vi "shag_start — 4.vi"() -> ()   [LabVIEW 2016]
uses:
  <vilib>/Instr/_visa.llb/VISA Configure Serial Port (Instr).vi
panel:
  out "положение в мин 1":i32
  in  "stop":bool
  in  "all":T1(tab)
  out "положение шд":i32(knob) scale=-10.0..190.0
  out "текущее положение":string
  out "положение в минутах 1":string
  in  "Минуты":i32 min=-600 max=11400
  in  "Stop двигатель":bool
  in  "Вращение по градусам +":bool
  in  "Вращение по градусам -":bool
  in  "Вернуться в нулевое положение":bool
  in  "Задать текущее положение нулевым":bool
  in  "Установка минут":bool
  in  "Блокировать зеркало №1":bool
  in  "Выберете COM порт":refnum<visa-resource-name>="COM1"
  in  "Скорость обмена данными":u32(ring)=19200 items=["9600"=9600, "19200"=19200, "38400"=38400, "57600"=57600]
  in  "Число бит на символ":u16=8 min=5 max=8 step=1
  in  "Контроль чётности":enum16{"None", "Odd", "Even", "Mark", "Space"}(ring)
  in  "Стоповый бит":u16(ring)=10 items=["1.0"=10, "1.5"=15, "2.0"=20]
  in  "Контроль переполнения":u16(ring) items=["None"=0, "XON/XOFF"=1, "RTS/CTS"=2, "DTR/DSR"=4]
  # "1 - адресс 1 двигателя\n2 - адресс 2 двигателя\n$0MV\\01+   - запуск всех двигателей в положительном направлении \n$0MS\\00   - остановка всех двигателей\n$0MJ\\04+\\00\\00\\01   - 1 шаг всех двигателей\n$0SS\\01\\10   - скорость 10 для всех двигателей"
  # "Зеркало №1:"
  # "Положение:"
  # "Ренгеновская трубка №2:"
  # "Положение ренгеновской трубк:"
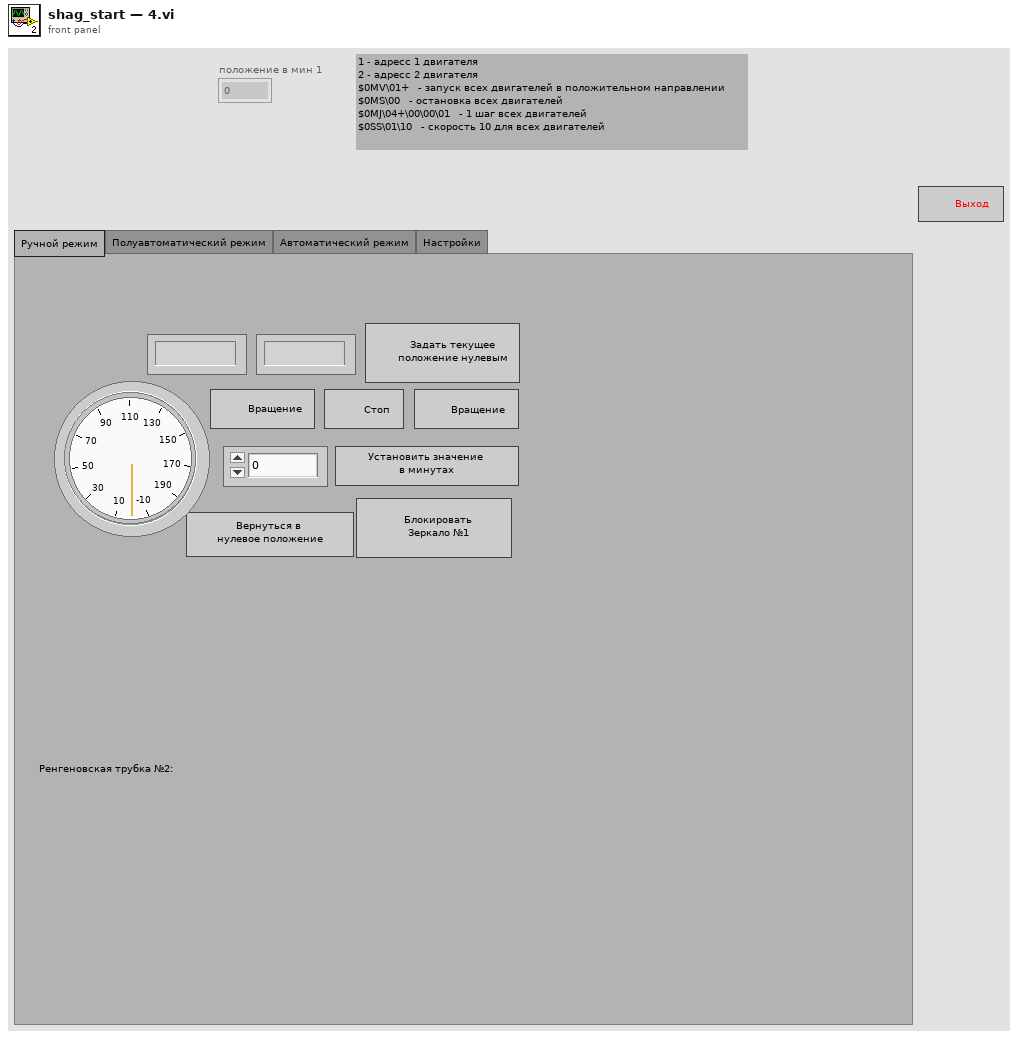
[diagram p1: front panel]
types:
  T1 = enum32{"Ручной режим", "Полуавтоматический режим", "Автоматический режим", "Настройки"}
  T2 = enum8{"Enabled", "Disabled", "Disabled and Grayed Out"}
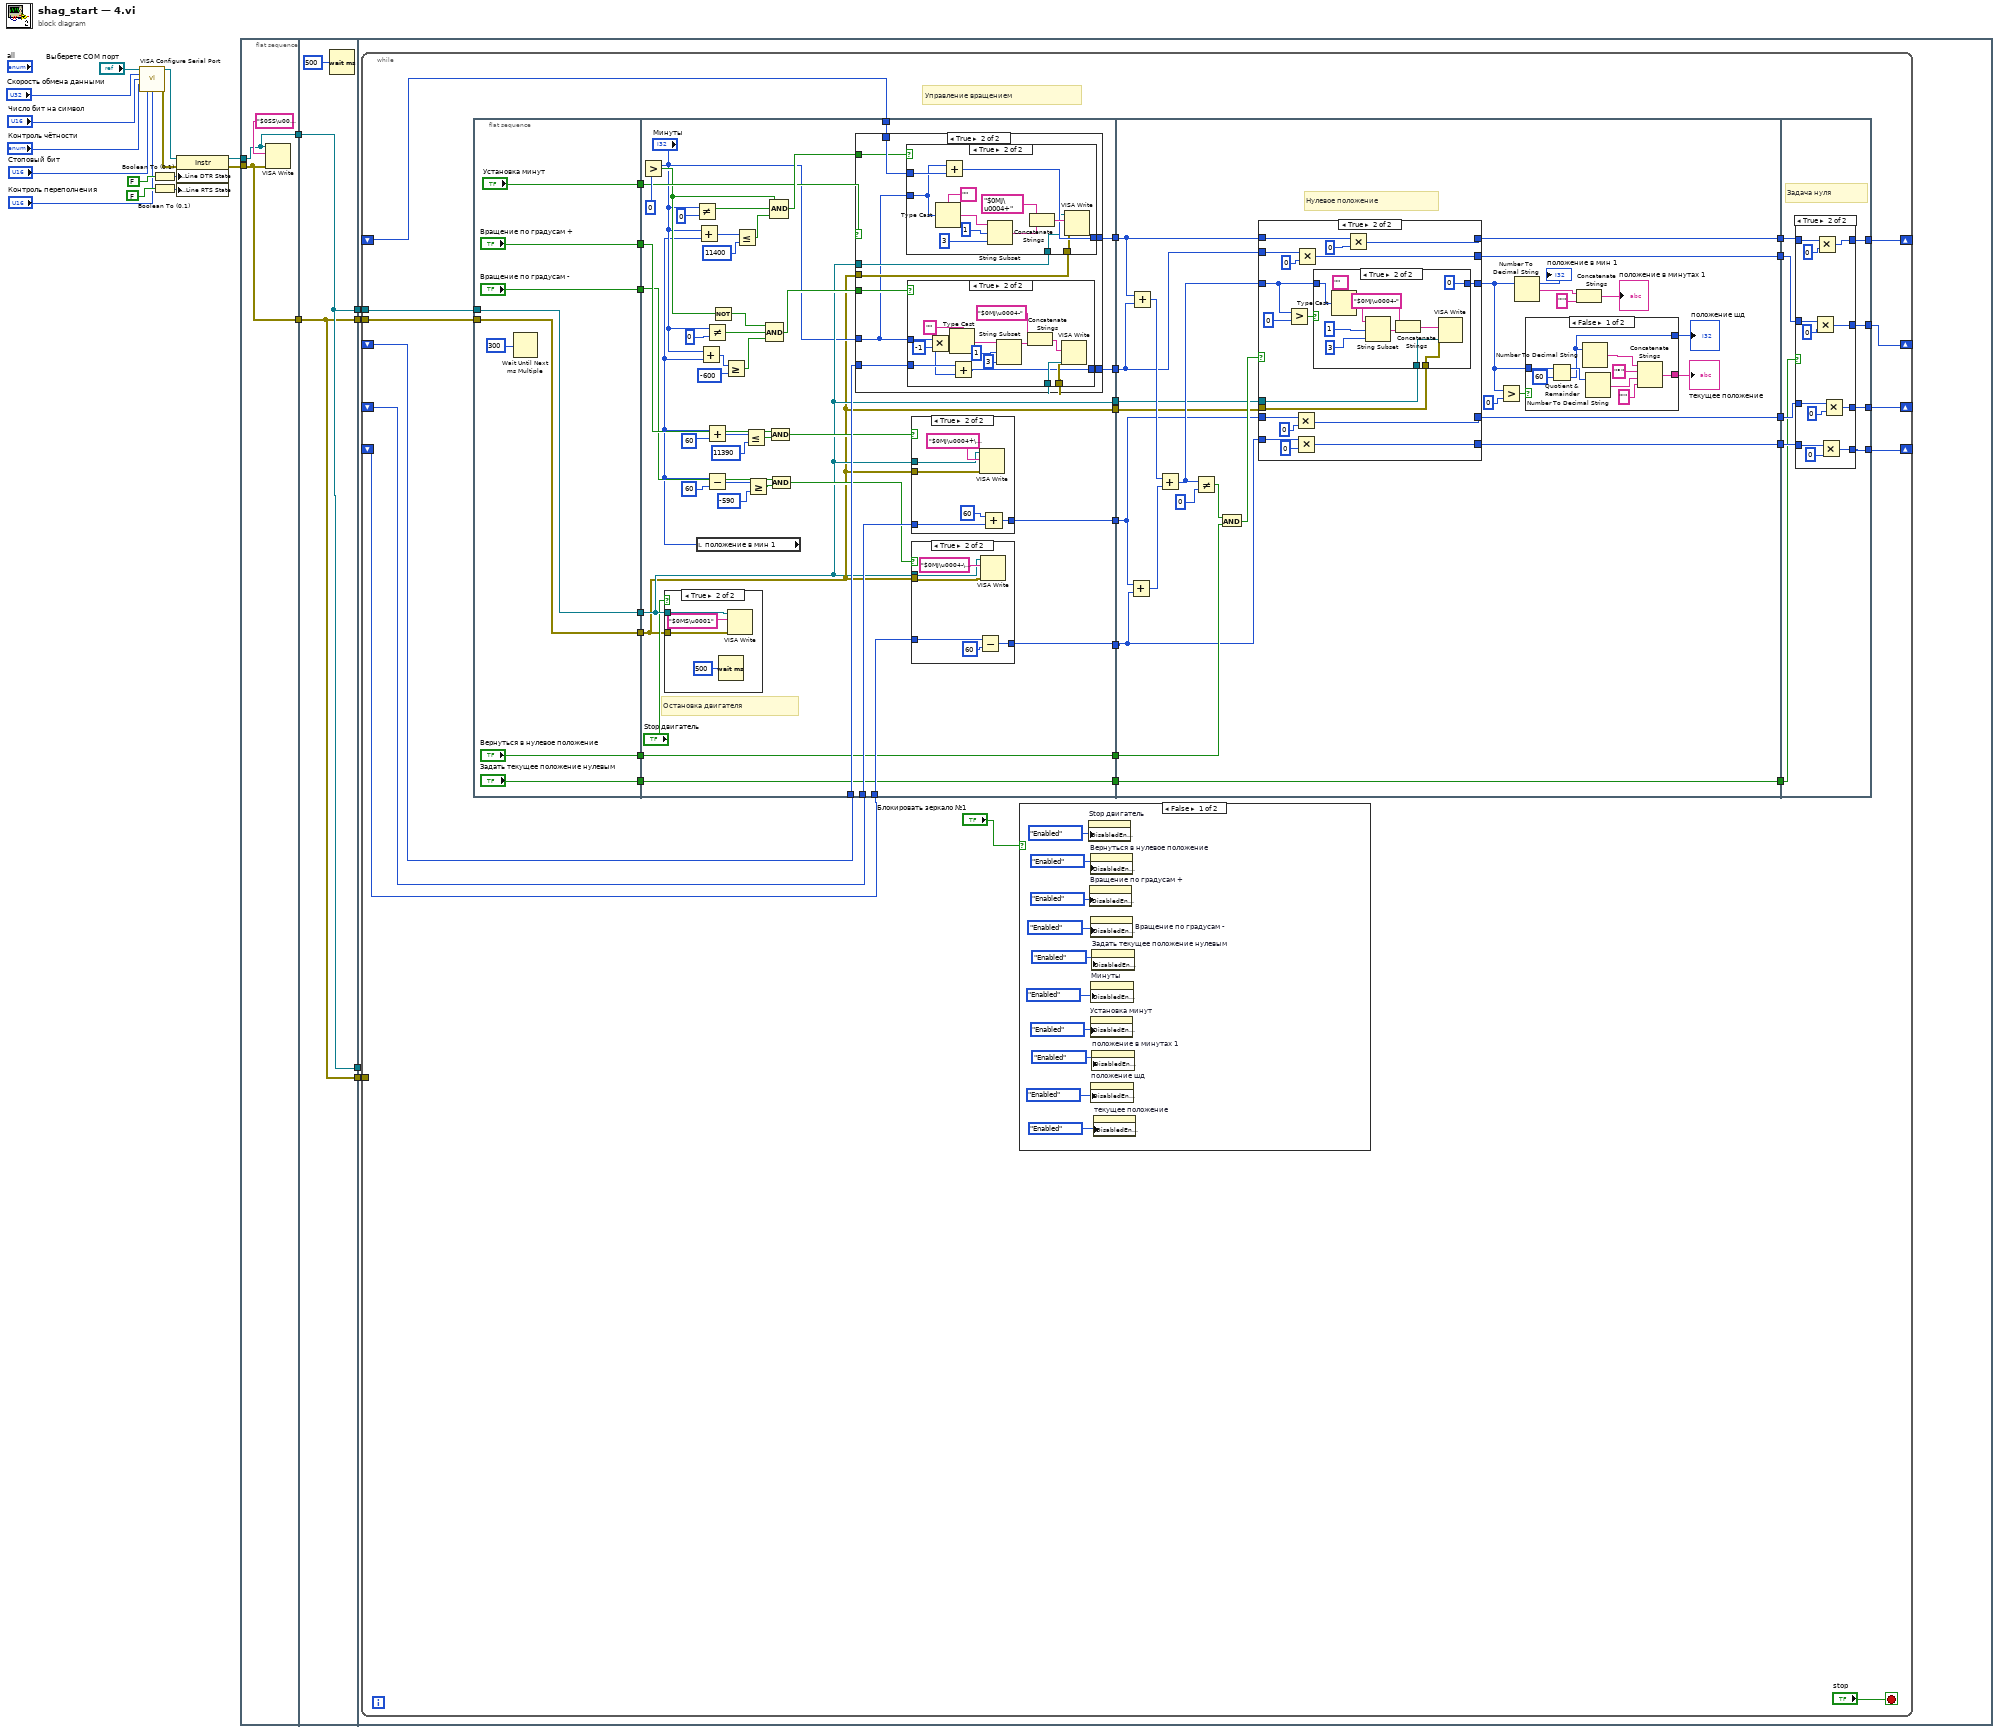
[diagram p0: block diagram]
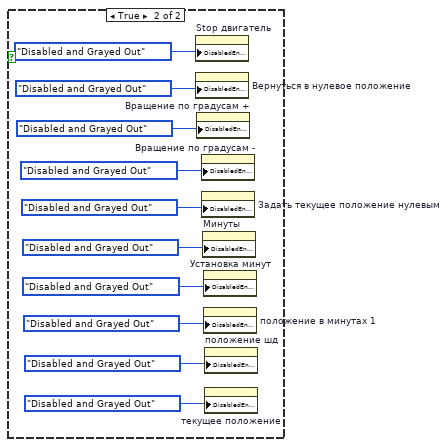
[diagram p2: hidden frame]
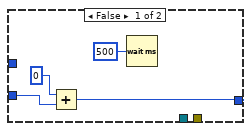
[diagram p4: hidden frame]
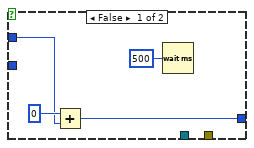
[diagram p5: hidden frame]
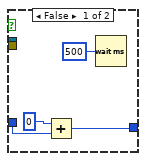
[diagram p7: hidden frame]
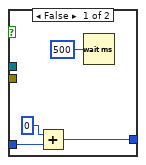
[diagram p8: hidden frame]
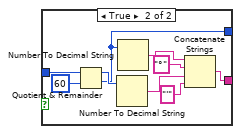
[diagram p9: hidden frame]
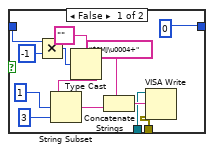
[diagram p11: hidden frame]
diagram:
  n1 = call-poly "VISA Configure Serial Port"("VISA resource name"="Выберете COM порт", "baud rate (9600)"="Скорость обмена данными", "data bits (8)"="Число бит на символ", "parity (0:none)"="Контроль чётности", "stop bits (10: 1 bit)"="Стоповый бит", "flow control (0:none)"="Контроль переполнения") -> ("VISA resource name out"=w18:refnum<visa-resource-name>, "error out"=w17:errorcluster)  [unwired: 8 in]
  n2 = Boolean To (0,1)(Boolean=FALSE ("DTR Write")) -> (0, 1=w19:i16)
  n3 = Boolean To (0,1)(Boolean=FALSE ("DTR Write")) -> (0, 1=w20:i16)
  n4 = property class="Instr"(reference=w18, error in=w17, "Serial Settings:Modem Line Settings:Line DTR State"=w19, "Serial Settings:Modem Line Settings:Line RTS State"=w20) -> (reference out=w16:refnum<visa-resource-name>, error out=w15:errorcluster)
  n5 = flat-sequence {
    tunnel: w16 -> [w22]
    tunnel: w15 -> [w21]
    tunnel: [w22] -> w13
    tunnel: [w21] -> w12
    tunnel: [w25] -> w14
    tunnel: w13 -> [w25]
    tunnel: w12 -> [w24]
    tunnel: [w24] -> w11
    tunnel: [w25] -> w2
    tunnel: [w24] -> w1
    tunnel: w14 -> [w29]
    tunnel: w11 -> [w28]
    tunnel: w2 -> [_]
    tunnel: w1 -> [w27]
    frame #0 {
      n6 = VISA Write(VISA resource name=w22, write buffer="$0SS\u0001\u0010", error in (no error)=w21) -> ()  [unwired: 3 out]
    }
    frame #1 {
      n7 = Wait (ms)(milliseconds to wait=u32 500) -> ()  [unwired: 1 out]
    }
    frame #2 {
      n8 = while {
        tunnel: w29 -> [w36]
        tunnel: w28 -> [w35]
        shift-right: [w31] -> _
        shift-left: _ -> [w40]
        shift-right: [w32] -> _
        shift-left: _ -> [w39]
        shift-right: [w33] -> _
        shift-left: _ -> [w38]
        shift-right: [w34] -> _
        shift-left: _ -> [w37]
        tunnel: w27 -> [_]
        stop <- "stop" stop-if-true
        # "Управление вращением"
        n9 = flat-sequence {
          tunnel: w35 -> [w88]
          tunnel: w36 -> [w89]
          tunnel: [w89] -> w60
          tunnel: [w88] -> w59
          tunnel: ["Вращение по градусам +"] -> w58
          tunnel: ["Вращение по градусам -"] -> w57
          tunnel: ["Вернуться в нулевое положение"] -> w56
          tunnel: ["Задать текущее положение нулевым"] -> w55
          tunnel: ["Установка минут"] -> w54
          tunnel: w60 -> [w109]
          tunnel: w59 -> [w90]
          tunnel: [w132] -> w53
          tunnel: w40 -> [w129]
          tunnel: w39 -> [w131]
          tunnel: [w130] -> w52
          tunnel: w38 -> [w128]
          tunnel: w37 -> [w127]
          tunnel: w58 -> [w113]
          tunnel: w57 -> [w112]
          tunnel: [w126] -> w51
          tunnel: [w125] -> w50
          tunnel: [w110] -> w49
          tunnel: w56 -> [w110]
          tunnel: [w90] -> w48
          tunnel: [w109] -> w47
          tunnel: [w108] -> w46
          tunnel: w55 -> [w108]
          tunnel: w54 -> [w102]
          tunnel: w53 -> [w206]
          tunnel: w52 -> [w207]
          tunnel: [w227] -> w45
          tunnel: [w225] -> w44
          tunnel: w51 -> [w208]
          tunnel: w50 -> [w209]
          tunnel: [w215] -> w43
          tunnel: [w223] -> w42
          tunnel: w49 -> [w219]
          tunnel: w48 -> [w214]
          tunnel: w47 -> [w213]
          tunnel: w46 -> [w211]
          tunnel: [w211] -> w41
          tunnel: [w301] -> w31
          tunnel: [w298] -> w32
          tunnel: w45 -> [w300]
          tunnel: w44 -> [w299]
          tunnel: [w297] -> w33
          tunnel: [w296] -> w34
          tunnel: w43 -> [w295]
          tunnel: w42 -> [w294]
          tunnel: w41 -> [w293]
          frame #0 {
            n10 = Wait Until Next ms Multiple(millisecond multiple=u32 300) -> ()  [unwired: 1 out]
          }
          frame #1 {
            # "Остановка двигателя"
            n11 = Greater?(x="Минуты", y=0) -> (0:w100:bool)
            n12 = case shown="True" "Stop двигатель" {
              tunnel: w109 -> [_ w179]
              tunnel: w90 -> [_ w178]
              frame False {
              }
              frame True {
                n13 = Wait (ms)(milliseconds to wait=u32 500) -> ()  [unwired: 1 out]
                n14 = VISA Write(VISA resource name=w179, write buffer="$0MS\u0001", error in (no error)=w178) -> ()  [unwired: 3 out]
              }
            }
            n15 = Not Equal?(x="Минуты", y=0) -> (x != y?=w99:bool)
            n16 = local read "положение в мин 1"() -> (w95:i32)
            n17 = Add(x="Минуты", y=w95) -> (x+y=w123:i32)
            n18 = Add(x="Минуты", y=w95) -> (x+y=w93:i32)
            n19 = Not Equal?(x="Минуты", y=0) -> (x != y?=w97:bool)
            n20 = Add(x=w95, y=60) -> (x+y=w118:i32)
            n21 = Subtract(x=w95, y=60) -> (x-y=w105:i32)
            n22 = Not(x=w100) -> (.not. x?=w101:bool)
            n23 = Greater Or Equal?(x=w93, y=-600) -> (x >= y?=w94:bool)
            n24 = Less Or Equal?(x=w123, y=11400) -> (x <= y?=w98:bool)
            n25 = Less Or Equal?(x=w118, y=11390) -> (x <= y?=w115:bool)
            n26 = Greater Or Equal?(x=w105, y=-590) -> (x >= y?=w106:bool)
            n27 = Compound Arithmetic op=AND(w101, w97, w94) -> (w119:bool)
            n28 = And(x=w113, y=w115) -> (x .and. y?=w114:bool)
            n29 = And(x=w112, y=w106) -> (x .and. y?=w111:bool)
            n30 = Compound Arithmetic op=AND(w100, w99, w98) -> (w121:bool)
            n31 = case shown="True" w102 {
              tunnel: [w134 w143] -> w132
              tunnel: w131 -> [w133 w142]
              tunnel: [w133 w141] -> w130
              tunnel: w129 -> [w134 w140]
              tunnel: w121 -> [_ w139]
              tunnel: w119 -> [_ w138]
              tunnel: w90 -> [_ w137]
              tunnel: w109 -> [_ w136]
              tunnel: "Минуты" -> [_ w135]
              frame False {
              }
              frame True {
                n32 = case shown="True" w139 {
                  tunnel: [w164 w170] -> w143
                  tunnel: w140 -> [w163 w169]
                  tunnel: w137 -> [_ w168]
                  tunnel: w136 -> [_ w167]
                  tunnel: w135 -> [_ w166]
                  frame False {
                    n33 = Add(x=0, y=w163) -> (x+y=w164:i32)
                    n34 = Wait (ms)(milliseconds to wait=u32 500) -> ()  [unwired: 1 out]
                  }
                  frame True {
                    n35 = Type Cast(type="", x=w166) -> (*(type *) &x=w173:string)
                    n36 = Add(x=w166, y=w169) -> (x+y=w170:i32)
                    n37 = String Subset(string=w173, offset (0)=1, length (rest)=3 ("length (rest)")) -> (substring=w172:string)
                    n38 = Concatenate Strings("$0MJ\u0004+" ("write buffer"), w172) -> (w176:string)
                    n39 = VISA Write(VISA resource name=w167, write buffer=w176, error in (no error)=w168) -> ()  [unwired: 3 out]
                  }
                }
                n40 = case shown="True" w138 {
                  tunnel: [w146 w152] -> w141
                  tunnel: w142 -> [w145 w151]
                  tunnel: w136 -> [_ w154]
                  tunnel: w137 -> [_ w153]
                  tunnel: w135 -> [_ w148]
                  frame False {
                    n41 = Add(x=0, y=w145) -> (x+y=w146:i32)
                    n42 = Wait (ms)(milliseconds to wait=u32 500) -> ()  [unwired: 1 out]
                  }
                  frame True {
                    n43 = Multiply(x=w148, y=-1) -> (x*y=w150:i32)
                    n44 = Type Cast(type="", x=w150) -> (*(type *) &x=w157:string)
                    n45 = Add(x=w151, y=w148) -> (x+y=w152:i32)
                    n46 = String Subset(string=w157, offset (0)=1, length (rest)=3 ("length (rest)")) -> (substring=w156:string)
                    n47 = Concatenate Strings("$0MJ\u0004-" ("write buffer"), w156) -> (w160:string)
                    n48 = VISA Write(VISA resource name=w154, write buffer=w160, error in (no error)=w153) -> ()  [unwired: 3 out]
                  }
                }
              }
            }
            n49 = case shown="True" w114 {
              tunnel: [w194 w201] -> w126
              tunnel: w128 -> [w193 w196]
              tunnel: w109 -> [_ w197]
              tunnel: w90 -> [_ w198]
              frame False {
                n50 = Add(x=0, y=w193) -> (x+y=w194:i32)
                n51 = Wait (ms)(milliseconds to wait=u32 500) -> ()  [unwired: 1 out]
              }
              frame True {
                n52 = VISA Write(VISA resource name=w197, write buffer="$0MJ\u0004+\u0000\u0000<", error in (no error)=w198) -> ()  [unwired: 3 out]
                n53 = Add(x=60, y=w196) -> (x+y=w201:i32)
              }
            }
            n54 = case shown="True" w111 {
              tunnel: [w184 w187] -> w125
              tunnel: w127 -> [w183 w186]
              tunnel: w109 -> [_ w190]
              tunnel: w90 -> [_ w189]
              frame False {
                n55 = Add(x=0, y=w183) -> (x+y=w184:i32)
                n56 = Wait (ms)(milliseconds to wait=u32 500) -> ()  [unwired: 1 out]
              }
              frame True {
                n57 = Subtract(x=w186, y=60 ("x")) -> (x-y=w187:i32)
                n58 = VISA Write(VISA resource name=w190, write buffer="$0MJ\u0004-\u0000\u0000<", error in (no error)=w189) -> ()  [unwired: 3 out]
              }
            }
          }
          frame #2 {
            # "Нулевое положение"
            n59 = Add(x=w208, y=w209) -> (x+y=w220:i32)
            n60 = Add(x=w206, y=w207) -> (x+y=w224:i32)
            n61 = Add(x=w224, y=w220) -> (x+y=w217:i32)
            n62 = Not Equal?(x=w217, y=0 ("x")) -> (x != y?=w216:bool)
            n63 = And(x=w216, y=w219) -> (x .and. y?=w226:bool)
            n64 = case shown="True" w226 {
              tunnel: [w248 w268] -> w205
              tunnel: w206 -> [w250 w265]
              tunnel: [w250 w264] -> w227
              tunnel: [w249 w263] -> w225
              tunnel: w217 -> [w248 w257]
              tunnel: [w246 w259] -> w223
              tunnel: [w247 w256] -> w215
              tunnel: w207 -> [w249 w255]
              tunnel: w214 -> [_ w254]
              tunnel: w213 -> [_ w253]
              tunnel: w208 -> [w247 w252]
              tunnel: w209 -> [w246 w251]
              frame False {
              }
              frame True {
                n65 = Greater?(x=w257, y=0) -> (0:w258:bool)
                n66 = Multiply(x=w252, y=0) -> (x*y=w256:i32)
                n67 = Multiply(x=w251, y=0) -> (x*y=w259:i32)
                n68 = Multiply(x=w255, y=0) -> (x*y=w263:i32)
                n69 = case shown="True" w258 {
                  tunnel: w257 -> [w273 w286]
                  tunnel: [0 0] -> w268
                  tunnel: w253 -> [w270 w283]
                  tunnel: w254 -> [w269 w282]
                  frame False {
                    n70 = Multiply(x=w273, y=-1) -> (x*y=w271:i32)
                    n71 = Type Cast(type="", x=w271) -> (*(type *) &x=w277:string)
                    n72 = String Subset(string=w277, offset (0)=1, length (rest)=3 ("length (rest)")) -> (substring=w276:string)
                    n73 = Concatenate Strings("$0MJ\u0004+" ("write buffer"), w276) -> (w280:string)
                    n74 = VISA Write(VISA resource name=w270, write buffer=w280, error in (no error)=w269) -> ()  [unwired: 3 out]
                  }
                  frame True {
                    n75 = Type Cast(type="", x=w286) -> (*(type *) &x=w289:string)
                    n76 = String Subset(string=w289, offset (0)=1, length (rest)=3 ("length (rest)")) -> (substring=w288:string)
                    n77 = Concatenate Strings("$0MJ\u0004-" ("write buffer"), w288) -> (w284:string)
                    n78 = VISA Write(VISA resource name=w283, write buffer=w284, error in (no error)=w282) -> ()  [unwired: 3 out]
                  }
                }
                n79 = Multiply(x=w265, y=0) -> (x*y=w264:i32)
              }
            }
            "положение в мин 1" <- w205
            n80 = Greater?(x=w205, y=0) -> (0:w222:bool)
            n81 = Number To Decimal String(number=w205) -> (decimal integer string=w203:string)  [unwired: 1 in]
            n82 = case shown="False" w222 {
              tunnel: w205 -> [w235 w245]
              tunnel: [w232 w239] -> w212
              tunnel: [w228 w237] -> w210
              frame False {
                n83 = Quotient & Remainder(x=w235, y=60) -> (x-y*floor(x/y)=w231:i32, floor(x/y)=w228:i32)
                n84 = Number To Decimal String(number=w228) -> (decimal integer string=w229:string)  [unwired: 1 in]
                n85 = Number To Decimal String(number=w231) -> (decimal integer string=w230:string)  [unwired: 1 in]
                n86 = Concatenate Strings(w229, "°" ("string"), w230, "'" ("string")) -> (w232:string)
              }
              frame True {
                n87 = Quotient & Remainder(x=w245, y=60) -> (x-y*floor(x/y)=w238:i32, floor(x/y)=w237:i32)
                n88 = Number To Decimal String(number=w238) -> (decimal integer string=w240:string)  [unwired: 1 in]
                n89 = Number To Decimal String(number=w237) -> (decimal integer string=w241:string)  [unwired: 1 in]
                n90 = Concatenate Strings(w241, "°" ("string"), w240, "'" ("string")) -> (w239:string)
              }
            }
            "положение шд" <- w210
            "текущее положение" <- w212
            n91 = Concatenate Strings(w203, "'" ("string")) -> (→"положение в минутах 1":string)
          }
          frame #3 {
            # "Задача нуля"
            n92 = case shown="True" w293 {
              tunnel: [w305 w316] -> w301
              tunnel: w300 -> [w305 w317]
              tunnel: w299 -> [w304 w313]
              tunnel: [w304 w312] -> w298
              tunnel: [w303 w309] -> w297
              tunnel: [w302 w308] -> w296
              tunnel: w295 -> [w303 w307]
              tunnel: w294 -> [w302 w306]
              frame False {
              }
              frame True {
                n93 = Multiply(x=w313, y=0) -> (x*y=w312:i32)
                n94 = Multiply(x=w317, y=0) -> (x*y=w316:i32)
                n95 = Multiply(x=w306, y=0) -> (x*y=w308:i32)
                n96 = Multiply(x=w307, y=0) -> (x*y=w309:i32)
              }
            }
          }
        }
        n97 = case shown="False" "Блокировать зеркало №1" {
          frame False {
            n98 = property on="Stop двигатель" class="Bool"("DisabledEnum"=T2."Enabled" ("Disabled")) -> ()  [unwired: 2 in, 2 out]
            n99 = property on="Вращение по градусам +" class="Bool"("DisabledEnum"=T2."Enabled" ("Disabled")) -> ()  [unwired: 2 in, 2 out]
            n100 = property on="Вернуться в нулевое положение" class="Bool"("DisabledEnum"=T2."Enabled" ("Disabled")) -> ()  [unwired: 2 in, 2 out]
            n101 = property on="Вращение по градусам -" class="Bool"("DisabledEnum"=T2."Enabled" ("Disabled")) -> ()  [unwired: 2 in, 2 out]
            n102 = property on="Установка минут" class="Bool"("DisabledEnum"=T2."Enabled" ("Disabled")) -> ()  [unwired: 2 in, 2 out]
            n103 = property on="Минуты" class="DigNum (strict)"("DisabledEnum"=T2."Enabled" ("Disabled")) -> ()  [unwired: 2 in, 2 out]
            n104 = property on="положение шд" class="Knob (strict)"("DisabledEnum"=T2."Enabled" ("Disabled")) -> ()  [unwired: 2 in, 2 out]
            n105 = property on="Задать текущее положение нулевым" class="Bool"("DisabledEnum"=T2."Enabled" ("Disabled")) -> ()  [unwired: 2 in, 2 out]
            n106 = property on="положение в минутах 1" class="Str"("DisabledEnum"=T2."Enabled" ("Disabled")) -> ()  [unwired: 2 in, 2 out]
            n107 = property on="текущее положение" class="Str"("DisabledEnum"=T2."Enabled" ("Disabled")) -> ()  [unwired: 2 in, 2 out]
          }
          frame True {
            n108 = property on="Stop двигатель" class="Bool"("DisabledEnum"=T2."Disabled and Grayed Out" ("Disabled")) -> ()  [unwired: 2 in, 2 out]
            n109 = property on="Вернуться в нулевое положение" class="Bool"("DisabledEnum"=T2."Disabled and Grayed Out" ("Disabled")) -> ()  [unwired: 2 in, 2 out]
            n110 = property on="Вращение по градусам +" class="Bool"("DisabledEnum"=T2."Disabled and Grayed Out" ("Disabled")) -> ()  [unwired: 2 in, 2 out]
            n111 = property on="Вращение по градусам -" class="Bool"("DisabledEnum"=T2."Disabled and Grayed Out" ("Disabled")) -> ()  [unwired: 2 in, 2 out]
            n112 = property on="Задать текущее положение нулевым" class="Bool"("DisabledEnum"=T2."Disabled and Grayed Out" ("Disabled")) -> ()  [unwired: 2 in, 2 out]
            n113 = property on="Минуты" class="DigNum (strict)"("DisabledEnum"=T2."Disabled and Grayed Out" ("Disabled")) -> ()  [unwired: 2 in, 2 out]
            n114 = property on="Установка минут" class="Bool"("DisabledEnum"=T2."Disabled and Grayed Out" ("Disabled")) -> ()  [unwired: 2 in, 2 out]
            n115 = property on="положение в минутах 1" class="Str"("DisabledEnum"=T2."Disabled and Grayed Out" ("Disabled")) -> ()  [unwired: 2 in, 2 out]
            n116 = property on="положение шд" class="Knob (strict)"("DisabledEnum"=T2."Disabled and Grayed Out" ("Disabled")) -> ()  [unwired: 2 in, 2 out]
            n117 = property on="текущее положение" class="Str"("DisabledEnum"=T2."Disabled and Grayed Out" ("Disabled")) -> ()  [unwired: 2 in, 2 out]
          }
        }
      }
    }
  }
